vi "Exclude_OK.vi"(3 "Exclude Array":T1[](array[typedef]) {"Sizes"."Min" format="%#.1f"; "Sizes"."Max" format="%#.1f"}, 4 "Previous Probe Volume":cluster{"Max":dbl, "Min":dbl}[](array[cluster]) {"Min" format="%.2f"; "Max" format="%.2f"}, 5 "Traverse Name":string, 6 "Probe Volume":cluster{"Max":dbl, "Min":dbl}[](array[cluster]) {"Min" format="%.2f"; "Max" format="%.2f"}) -> (0 "Error Comments":string, 1 "Separation Distance":dbl format="%.2f", 2 "Probe OK?":bool)   [LabVIEW 2010]
uses:
  Exclude_cluster.ctl
  Box_size.ctl
  Exclusion_type.ctl
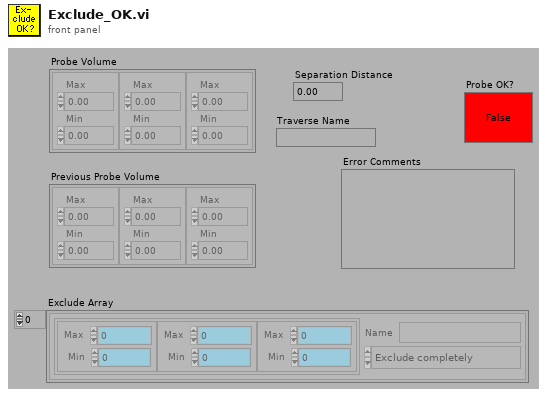
[diagram p1: front panel]
types:
  T1 = typedef "Exclude_cluster.ctl" = cluster{"Sizes":T2, "Name":string, "Exclude Type":T3}
  T2 = typedef "Box_size.ctl" = cluster{"Max":dbl, "Min":dbl}[]
  T3 = typedef "Exclusion_type.ctl" = enum16{"Exclude completely", "Allow only vertical moves"}
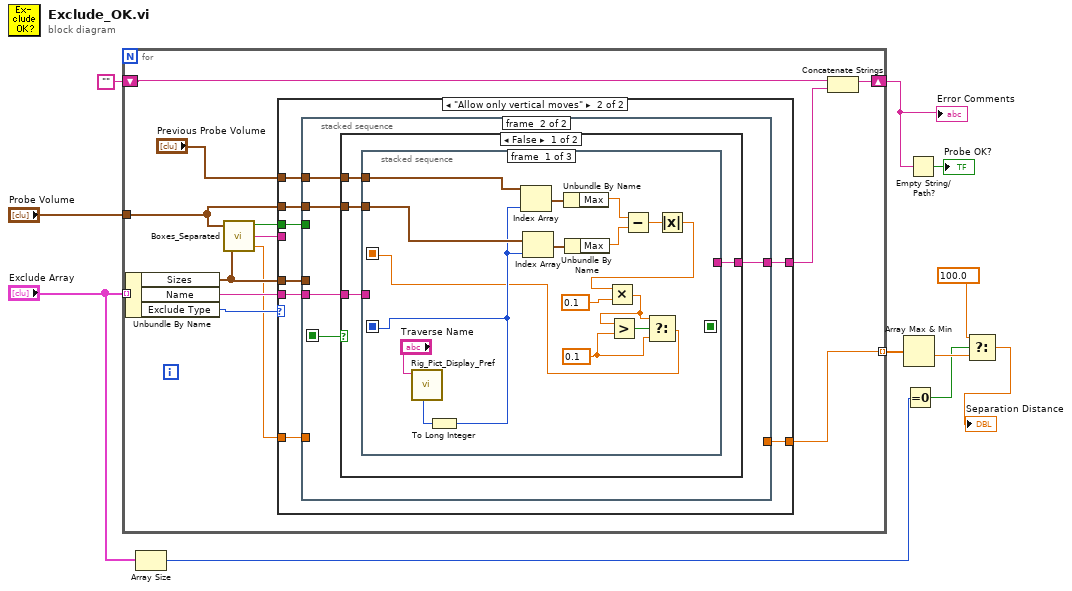
[diagram p0: block diagram]
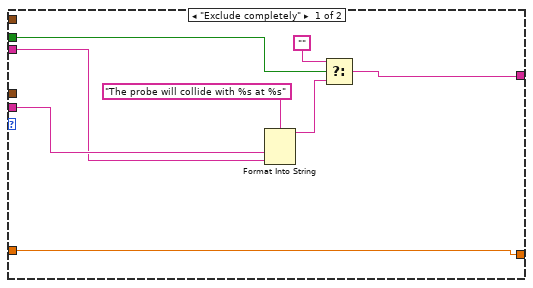
[diagram p2: hidden frame]
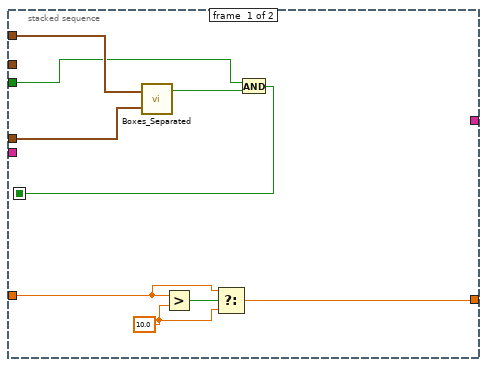
[diagram p3: hidden frame]
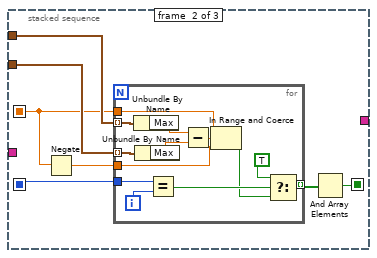
[diagram p4: hidden frame]
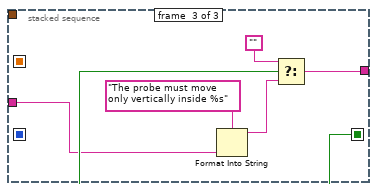
[diagram p5: hidden frame]
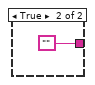
[diagram p6: hidden frame]
diagram:
  n1 = for {
    tunnel: "Exclude Array" -> [w24] mode=indexing
    tunnel: "Probe Volume" -> [w17]
    shift-right: [w18] -> w9
    shift-left: "" -> [w20]
    tunnel: [w12] -> w7 mode=indexing
    n2 = Unbundle By Name(w24) -> ("Sizes"=w15:T2, "Name"=w22:string, "Exclude Type"=w23:T3)
    n3 = call "Boxes_Separated.vi"("Box 1"=w17, "Box 2"=w15) -> ("Box Separated"=w21:bool, "Error String"=w14:string, "Separation Distance"=w13:dbl)
    n4 = case shown="\"Allow only vertical moves\"" w23 {
      tunnel: w22 -> [w31 w37]
      tunnel: w21 -> [w30 w40]
      tunnel: [w27 w39] -> w19
      tunnel: w17 -> [_ w38]
      tunnel: "Previous Probe Volume" -> [_ w36]
      tunnel: w15 -> [_ w35]
      tunnel: w14 -> [w26 _]
      tunnel: w13 -> [w25 w34]
      tunnel: [w25 w33] -> w12
      frame "Exclude completely" {
        n5 = Format Into String(format string="The probe will collide with %s at %s" ("Format String"), w31, w26) -> (resulting string=w29:string)  [unwired: 2 in, 1 out]
        n6 = Select(t="", s=w30, f=w29) -> (s? t:f=w27:string)
      }
      frame "Allow only vertical moves" {
        n7 = stacked-sequence {
          seq-local: [w45 _] -> [_ w50]
          tunnel: w40 -> [w46 _]
          tunnel: [_ w54] -> w39
          tunnel: w38 -> [_ w53]
          tunnel: w37 -> [_ w52]
          tunnel: w36 -> [w49 w51]
          tunnel: w35 -> [w48 _]
          tunnel: w34 -> [w43 _]
          tunnel: [w41 _] -> w33
          frame #0 {
            w42 = 10.0 ("y")
            n8 = call "Boxes_Separated.vi"("Box 1"=w49, "Box 2"=w48) -> ("Box Separated"=w47:bool)  [unwired: 2 out]
            n9 = Greater?(x=w43, y=w42) -> (0:w44:bool)
            n10 = Select(t=w43, s=w44, f=w42) -> (s? t:f=w41:dbl)
            n11 = And(x=w46, y=w47) -> (x .and. y?=w45:bool)
          }
          frame #1 {
            n12 = case shown="False" w50 {
              tunnel: [w56 ""] -> w54
              tunnel: w53 -> [w58 _]
              tunnel: w52 -> [w57 _]
              tunnel: w51 -> [w55 _]
              frame False {
                n13 = stacked-sequence {
                  seq-local: [_ w79 _] -> [_ _ w97]
                  seq-local: [w70 _ _] -> [_ w77 _]
                  seq-local: [w59 _ _] -> [_ w76 _]
                  tunnel: w58 -> [w71 w81 _]
                  tunnel: w57 -> [_ _ w96]
                  tunnel: [_ _ w95] -> w56
                  tunnel: w55 -> [w72 w78 _]
                  frame #0 {
                    w60 = 0.1 ("y")
                    n14 = call "Rig_Pict_Display_Pref.vi"("Traverse Name"="Traverse Name") -> ("Which Axis is vertical?"=w74:enum16{"X Axis", "Y Axis", "Z Axis"})  [unwired: 7 out]
                    n15 = To Long Integer(number=w74) -> (32bit integer=w70:i32)
                    n16 = Index Array(array=w72, index=w70) -> (element=w69:cluster{"Max":dbl, "Min":dbl})
                    n17 = Index Array(array=w71, index=w70) -> (element=w68:cluster{"Max":dbl, "Min":dbl})
                    n18 = Unbundle By Name(w69) -> ("Max"=w67:dbl)
                    n19 = Unbundle By Name(w68) -> ("Max"=w66:dbl)
                    n20 = Subtract(x=w67, y=w66) -> (x-y=w65:dbl)
                    n21 = Absolute Value(x=w65) -> (abs(x)=w64:dbl)
                    n22 = Multiply(x=w64, y=0.1) -> (x*y=w61:dbl)
                    n23 = Greater?(x=w61, y=w60) -> (0:w62:bool)
                    n24 = Select(t=w61, s=w62, f=w60) -> (s? t:f=w59:dbl)
                  }
                  frame #1 {
                    n25 = Negate(x=w76) -> (-x=w75:dbl)
                    n26 = for {
                      tunnel: w78 -> [w94] mode=indexing
                      tunnel: w81 -> [w93] mode=indexing
                      tunnel: w77 -> [w92]
                      tunnel: [w88] -> w80 mode=indexing
                      tunnel: w76 -> [w83]
                      tunnel: w75 -> [w82]
                      i -> [w91]
                      n27 = Unbundle By Name(w94) -> ("Max"=w87:dbl)
                      n28 = Unbundle By Name(w93) -> ("Max"=w86:dbl)
                      n29 = Equal?(x=w92, y=w91) -> (x = y?=w90:bool)
                      n30 = Subtract(x=w87, y=w86) -> (x-y=w85:dbl)
                      n31 = In Range and Coerce(upper limit=w83, x=w85, lower limit=w82) -> (In Range?=w84:bool)  [unwired: 1 out]
                      n32 = Select(t=TRUE, s=w90, f=w84) -> (s? t:f=w88:bool)
                    }
                    n33 = And Array Elements(Boolean array=w80) -> (logical AND=w79:bool)
                  }
                  frame #2 {
                    n34 = Format Into String(format string="The probe must move only vertically inside %s" ("Format String"), w96) -> (resulting string=w99:string)  [unwired: 2 in, 1 out]
                    n35 = Select(t="", s=w97, f=w99) -> (s? t:f=w95:string)
                  }
                }
              }
              frame True {
              }
            }
          }
        }
      }
    }
    n36 = Concatenate Strings(w20, w19) -> (w18:string)
  }
  "Error Comments" <- w9
  n37 = Array Size(array="Exclude Array") -> (size(s)=w1:i32)
  n38 = Array Max & Min(array=w7) -> (min value=w6:dbl)  [unwired: 3 out]
  n39 = Equal To 0?(x=w1) -> (x = 0?=w5:bool)
  n40 = Empty String/Path?(string/path=w9) -> (empty?=→"Probe OK?":bool)
  n41 = Select(t=100.0, s=w5, f=w6) -> (s? t:f=→"Separation Distance":dbl)
